vi "TDT-Wait For DI Buffer Space.vi"(0 "RPcox":refnum<k7>, 5 "Next Buffer":i32, 7 "Tag":string="ch2Index", 9 "Buffer Length":i32, 11 "error in (no error)":errorcluster) -> (4 "RPcox Out":refnum<k7>, 6 "Next Buffer Out":i32, 15 "error out":errorcluster)   [LabVIEW 2020]
uses:
  TDT-Globals.vi
panel:
  in  "Timeout (ms)":i32=5000
  out "Available":bool
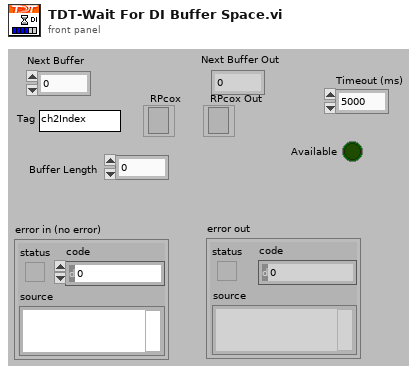
[diagram p1: front panel]
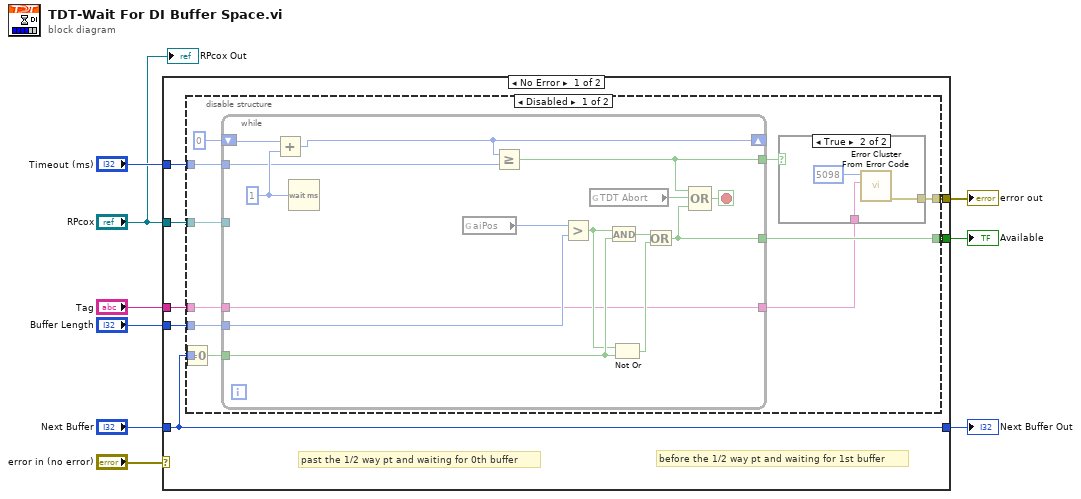
[diagram p0: block diagram]
diagram:
  n1 = case shown="No Error" "error in (no error)" {
    selector: "error in (no error)" -> [_ w46]
    tunnel: [w11 w46] -> w8
    tunnel: "Buffer Length" -> [w16 _]
    tunnel: "Next Buffer" -> [w14 _]
    tunnel: [w15 _] -> w5
    tunnel: [w14 _] -> w4
    tunnel: "Tag" -> [w13 _]
    tunnel: "Timeout (ms)" -> [w12 _]
    tunnel: "RPcox" -> [w10 _]
    frame No Error {
      # "before the 1/2 way pt and waiting for 1st buffer"
      # "past the 1/2 way pt and waiting for 0th buffer"
      n2 = disable-structure shown="Disabled" {
        disable-tunnel: w16 -> [w27 _]
        disable-tunnel: [w25 _] -> w15
        disable-tunnel: w14 -> [w24 _]
        disable-tunnel: w13 -> [w23 _]
        disable-tunnel: w12 -> [w21 _]
        disable-tunnel: [w18 _] -> w11
        disable-tunnel: w10 -> [w17 _]
        frame Disabled {
          n3 = Equal To 0?(x=w24) -> (x = 0?=w26:bool)
          n4 = while {
            tunnel: w27 -> [w33]
            tunnel: w26 -> [w44]
            tunnel: [w40] -> w25
            tunnel: w23 -> [w32]
            shift-right: [w36] -> _
            shift-left: 0 -> [w38]
            tunnel: w21 -> [w35]
            tunnel: [w34] -> w20
            tunnel: [w32] -> w19
            tunnel: w17 -> [_]
            stop <- w39 stop-if-true
            w37 = u32 1 ("milliseconds to wait")
            n5 = Add(x=w38, y=w37) -> (x+y=w36:u32)
            n6 = Wait (ms)(milliseconds to wait=w37) -> ()  [unwired: 1 out]
            n7 = global read "TDT-Globals.vi" "aiPos"() -> (w31:i32)
            n8 = Greater Or Equal?(x=w36, y=w35) -> (x >= y?=w34:bool)
            n9 = Greater?(x=w31, y=w33) -> (0:w43:bool)
            n10 = global read "TDT-Globals.vi" "TDT Abort"() -> (w41:bool)
            n11 = And(x=w43, y=w44) -> (x .and. y?=w45:bool)
            n12 = Not Or(1:w44, 2:w43) -> (0:w42:bool)
            n13 = Or(x=w45, y=w42) -> (x .or. y?=w40:bool)
            n14 = Compound Arithmetic op=OR(w34, w41, w40) -> (w39:bool)
          }
          n15 = case shown="True" w20 {
            tunnel: w19 -> [_ w29]
            tunnel: [_ w28] -> w18
            frame False {
            }
            frame True {
              n16 = call <vilib>:"Error Cluster From Error Code.vi"("error message (\"\")"=w29, "error code (0)"=5098 ("specific error code to clear (0: all)")) -> ("error out"=w28:errorcluster)  [unwired: 7 in]
            }
          }
        }
        frame Enabled {
        }
      }
    }
    frame Error {
    }
  }
  "error out" <- w8
  "Next Buffer Out" <- w4
  "Available" <- w5
  "RPcox Out" <- "RPcox"
